vi "Temp_to_Volt.vi"(1 "Temperature":dbl) -> (0 "Voltage":dbl)   [LabVIEW 2010]
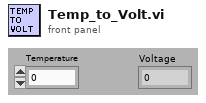
[diagram p1: front panel]
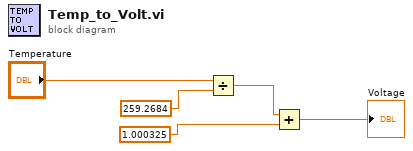
[diagram p0: block diagram]
diagram:
  n1 = Divide(x="Temperature", y=259.2684) -> (x/y=w2:dbl)
  n2 = Add(x=w2, y=1.000325) -> (x+y=→"Voltage":dbl)
